vi "data.vi"(10 "Numeric":i32=2121) -> (2 "Cluster":cluster{"Temperature":i32, "horodatage":string})   [LabVIEW 2014]
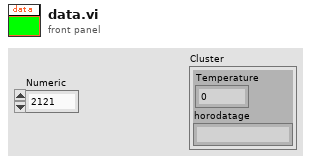
[diagram p1: front panel]
types:
  T1 = cluster{"Numeric":i32, "date/time string":string}
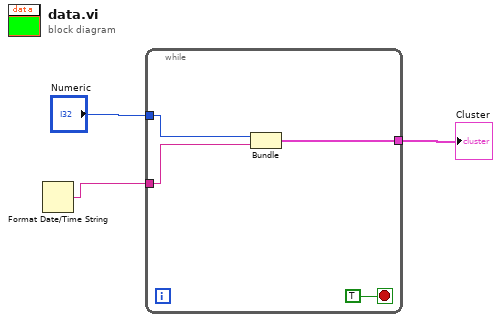
[diagram p0: block diagram]
diagram:
  n1 = Format Date/Time String() -> (date/time string=w2:string)  [unwired: 3 in]
  n2 = while {
    tunnel: "Numeric" -> [w6]
    tunnel: w2 -> [w5]
    tunnel: [w4] -> w1
    stop <- TRUE stop-if-true
    n3 = Bundle("Numeric"=w6, "date/time string"=w5) -> (w4:T1)  [unwired: 1 in]
  }
  "Cluster" <- w1
